vi "Add ROI Offset ImgData.vi"(4 "Region of Interest":i32[](array[numeric])=[-1, -1, 32000, 32000], 5 "ImgData In":T1={"X Intensity"=[], "Y Intensity"=[], "Max Intensity"=0.0, "Center"={"X"=0.0, "Y"=0.0}, "Radius"={"Rx"=239.10901, "Ry"=287.93375}}) -> (2 "ImgData Out":T1={"X Intensity"=[], "Y Intensity"=[], "Max Intensity"=0.0, "Center"={"X"=0.0, "Y"=0.0}, "Radius"={"Rx"=239.10901, "Ry"=287.93375}})   [LabVIEW 2013]
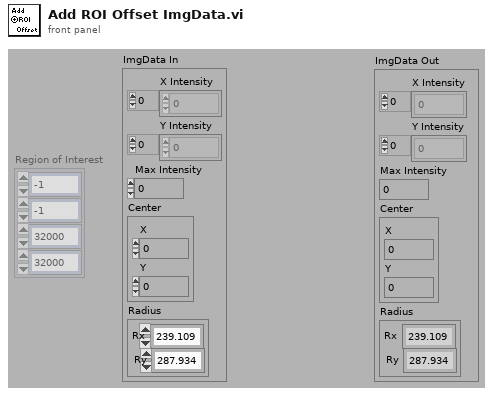
[diagram p1: front panel]
types:
  T1 = cluster{"X Intensity":u8[], "Y Intensity":u8[], "Max Intensity":sgl, "Center":cluster{"X":sgl, "Y":sgl}, "Radius":cluster{"Rx":sgl, "Ry":sgl}}
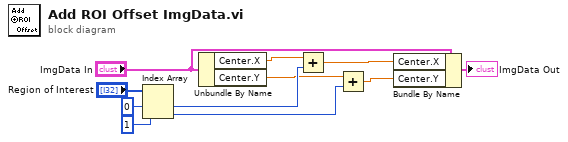
[diagram p0: block diagram]
diagram:
  n1 = Index Array(array="Region of Interest", index #1=0 ("index"), index #2=1 ("index")) -> (element #1=w8:i32, element #2=w7:i32)
  n2 = Unbundle By Name("ImgData In") -> ("Center.X"=w4:sgl, "Center.Y"=w6:sgl)
  n3 = Add(x=w4, y=w8) -> (x+y=w5:sgl)
  n4 = Add(x=w6, y=w7) -> (x+y=w3:sgl)
  n5 = Bundle By Name(cluster="ImgData In", "Center.X"=w5, "Center.Y"=w3) -> (→"ImgData Out":T1)
